vi "Initialize Starter Kit 2.0 from FPGA Refnum.vi"(8 "error in (no error)":errorcluster, 11 "FPGA refnum":refnum<k20>) -> (0 "error out":errorcluster, 3 "FPGA starter kit host out":refnum<class "NI_Robotics_Starter Kit Host_FPGA_2.0.lvclass">)   [LabVIEW 2017, in "NI_Robotics_Starter Kit Host_FPGA_2.0.lvclass"]
uses:
  <vilib>/robotics/Starter Kit/2.0/FPGA Host Interface/NI_Robotics_Starter Kit Host_FPGA_2.0.lvclass
  c:/Program Files (x86)/National Instruments/LabVIEW 2017/vi.lib/robotics/Starter Kit/Host Interface/NI_Robotics_Starter Kit Host.lvclass
  <vilib>/robotics/Starter Kit/2.0/FPGA Host Interface/FPGA Refnum.ctl
  <vilib>/robotics/Starter Kit/2.0/FPGA Host Interface/NI_Robotics_Starter Kit Host_FPGA_2.0.lvclass/NI_Robotics_Starter Kit Host_FPGA_2.0.ctl
  <vilib>/robotics/Starter Kit/Host Interface/NI_Robotics_Starter Kit Host.lvclass/NI_Robotics_Starter Kit Host.ctl
  <vilib>/robotics/Starter Kit/FPGA Direct IO/NI_Robotics_Starter Kit Direct IO_FPGA.lvclass/NI_Robotics_Starter Kit Direct IO_FPGA.ctl
  <vilib>/robotics/Starter Kit/Base Device/NI_Robotics_Starter Kit Base Device.lvclass/NI_Robotics_Starter Kit Base Device.ctl
  <vilib>/robotics/Starter Kit/Host Interface/Set DC Motors.vi
  <vilib>/robotics/Starter Kit/Host Interface/Set PING))) Sensor.vi
  <vilib>/robotics/Starter Kit/Host Interface/Set Sensor Servo.vi
  <vilib>/robotics/Starter Kit/FPGA Direct IO/Create FPGA Direct IO.vi
  <vilib>/robotics/Starter Kit/Host Interface/Set Direct IO.vi
  <vilib>/robotics/Starter Kit/Host Interface/Mark Initialized.vi
  <vilib>/robotics/Starter Kit/Base Device/Mark Initialized.vi
  <vilib>/robotics/Starter Kit/Servo Motor 2.0/NI_Robotics_Starter Kit Servo Motor_2.0.lvclass
  c:/Program Files (x86)/National Instruments/LabVIEW 2017/vi.lib/robotics/Starter Kit/Servo Motor/NI_Robotics_Starter Kit Servo Motor.lvclass
  <vilib>/robotics/Starter Kit/FPGA Direct IO/NI_Robotics_Starter Kit Direct IO_FPGA.lvclass
  c:/Program Files (x86)/National Instruments/LabVIEW 2017/vi.lib/robotics/Starter Kit/Base Device/NI_Robotics_Starter Kit Base Device.lvclass
  c:/Program Files (x86)/National Instruments/LabVIEW 2017/vi.lib/robotics/Starter Kit/Direct IO/NI_Robotics_Starter Kit Direct IO.lvclass
  <vilib>/robotics/Starter Kit/Servo Motor 2.0/Create 2.0 Servo Motor.vi
  <instrlib>/Hitec HS400 Series/HAIOL/FPGA/Public/Initialize (FPGA).vi
  <instrlib>/Parallax PING)))/HAIOL/FPGA/Public/Initialize (FPGA).vi
  <instrlib>/DC Motor Controller/HAIOL/FPGA/Public/Initialize (FPGA).vi
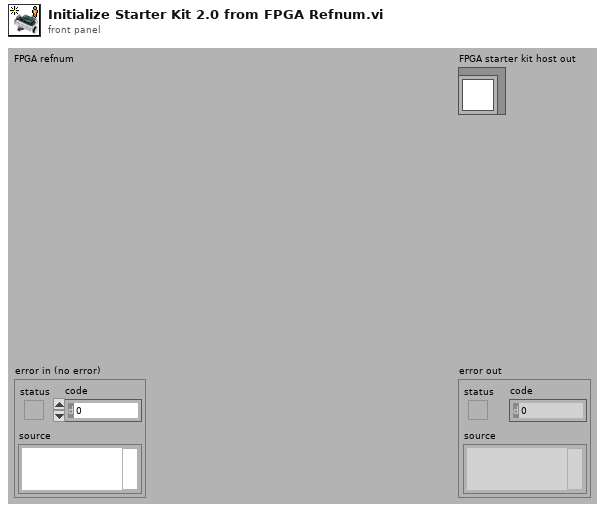
[diagram p1: front panel]
types:
  T1 = typedef "NI_Robotics_Starter Kit Host_FPGA_2.0.lvclass/FPGA Refnum.ctl" = refnum<k20>
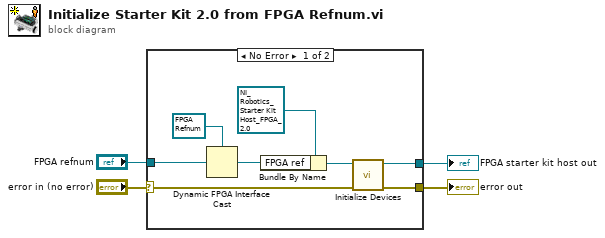
[diagram p0: block diagram]
diagram:
  n1 = case shown="No Error" "error in (no error)" {
    selector: "error in (no error)" -> [w6 w13]
    tunnel: [w5 w13] -> w3
    tunnel: "FPGA refnum" -> [w12 _]
    tunnel: [w7 _] -> w1
    frame No Error {
      n2 = Dynamic FPGA Interface Cast(Session In=T1 refnum ("FPGA ref"), Type=w12) -> (Session Out=w9:T1)
      n3 = Bundle By Name(cluster=refnum<class "NI_Robotics_Starter Kit Host_FPGA_2.0.lvclass"> refnum ("NI_Robotics_Starter Kit Host_FPGA_2.0.lvclass"), "FPGA ref"=w9) -> (w8:refnum<class "NI_Robotics_Starter Kit Host_FPGA_2.0.lvclass">)
      n4 = call <vilib>:"Initialize Devices.vi"("error in (no error)"=w6, "Starter Kit host FPGA 2.0 in"=w8) -> ("error out"=w5:errorcluster, "Starter Kit host FPGA 2.0 out"=w7:refnum<class "NI_Robotics_Starter Kit Host_FPGA_2.0.lvclass">)  [unwired: 8 in]
    }
    frame Error {
    }
  }
  "error out" <- w3
  "FPGA starter kit host out" <- w1
